vi "configcom.vi"(11 "Com port":i32=1 min=1 max=16 step=1) -> (0 "error out":errorcluster, 2 "Status":string, 3 "MSCU":refnum<class "MSCU.lvclass">)   [LabVIEW 2019, in "MSCU.lvclass"]
uses:
  MSCU.lvclass
  MSCU.lvclass/MSCU.ctl
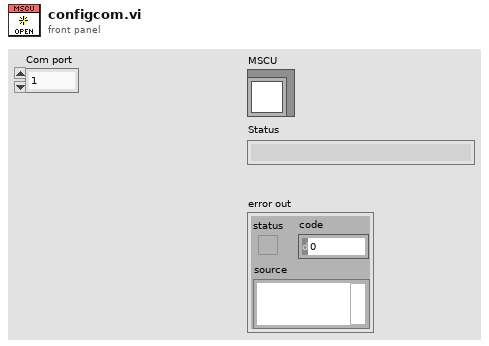
[diagram p1: front panel]
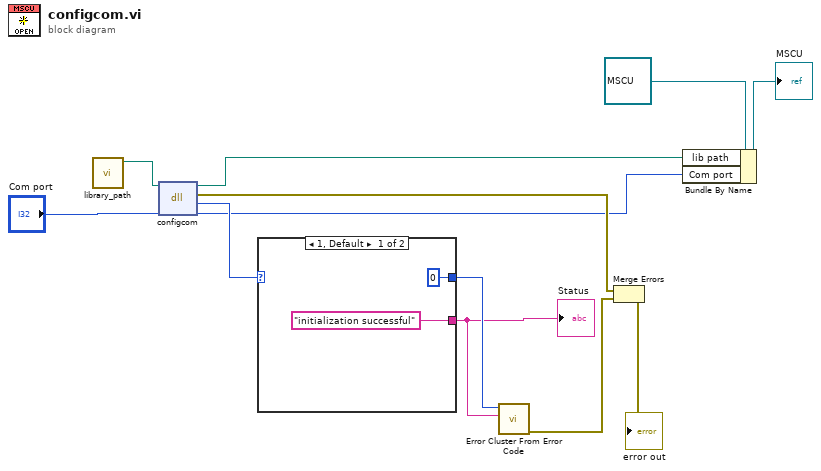
[diagram p0: block diagram]
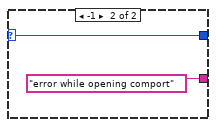
[diagram p2: hidden frame]
diagram:
  n1 = call "library_path.vi"() -> ("path out"=w3:path)  [unwired: 11 in]
  n2 = dll-call lib="C:/Program Files (x86)/Nanonis/SPM Controller/data/MSCU.dll" fn="configcom"(path in=w3, "Comport"="Com port") -> (path out=w2:path, error out=w8:errorcluster, "return type"=w12:i32, "Comport"=w4:i32)  [unwired: 2 in]
  n3 = case shown="1, Default" w12 {
    selector: w12 -> [_ w16]
    tunnel: ["initialization successful" "error while opening comport"] -> w9
    tunnel: [0 ("return type") w16] -> w11
    frame 1, Default {
    }
    frame -1 {
    }
  }
  "Status" <- w9
  n4 = call <vilib>:"Error Cluster From Error Code.vi"("error message (\"\")"=w9, "error code (0)"=w11) -> ("error out"=w7:errorcluster)  [unwired: 7 in]
  n5 = Merge Errors(w8, w7) -> (→"error out":errorcluster)
  n6 = Bundle By Name(cluster=refnum<class "MSCU.lvclass"> refnum ("MSCU.lvclass"), "lib path"=w2, "Com port"=w4) -> (→"MSCU":refnum<class "MSCU.lvclass">)
